vi "NEWER NEWEST Tilt Platform Controller.vi"() -> ()   [LabVIEW 2014]
uses:
  <vilib>/Utility/file.llb/Write To Spreadsheet File (DBL).vi
  <vilib>/Utility/file.llb/Read From Spreadsheet File (DBL).vi
  <vilib>/DAQmx/create/channels.llb/DAQmx Create Channel (DO-Digital Output).vi
  <vilib>/DAQmx/create/channels.llb/DAQmx Create Channel (AI-Voltage-Basic).vi
  <vilib>/DAQmx/configure/timing.llb/DAQmx Timing (Sample Clock).vi
  <vilib>/DAQmx/create/channels.llb/DAQmx Create Channel (DI-Digital Input).vi
  <vilib>/DAQmx/create/channels.llb/DAQmx Create Channel (CO-Pulse Generation-Ticks).vi
  <vilib>/DAQmx/configure/timing.llb/DAQmx Timing (Implicit).vi
  <vilib>/DAQmx/configure/trigger.llb/DAQmx Start Trigger (Digital Edge).vi
  <vilib>/DAQmx/read.llb/DAQmx Read (Analog 1D Wfm NChan NSamp).vi
  <vilib>/DAQmx/read.llb/DAQmx Read (Digital Wfm 1Chan NSamp).vi
  <vilib>/Waveform/DWDTOps.llb/DWDT Digital to Boolean Array.vi
  <vilib>/DAQmx/write.llb/DAQmx Write (Digital 1D Bool 1Chan 1Samp).vi
panel:
  out "In Position":bool
  in  "Divisor":u32=40
  in  "Signal Input":tag="/Dev3/PFI0"
  in  "Counter to Use":tag="Dev3/ctr0"
  in  "Start from Tilt":i32
  out "Ready":bool
  in  "Replay File":path=path "C:/Documents and Settings/theMaster/Desktop/Tilt Platform Control 9232015/Labview/Current_Tilts.csv"
  in  "Load Sequence":bool
  in  "Format":string="%.3f"
  in  "Delimiter":string=","
  in  "Column/Row Major":bool
  in  "Append to File?":bool=TRUE
  out "File Path":path
  out "Waveform Chart (Multiple Plots)":waveform(dbl)[](graph)
  in  "Callib Acce":bool
  in  "Callib Load Cell":bool
  in  "Transect?":bool
  in  "Week Number":dbl
  in  "Rat ID":string
  out "4":bool
  out "5":bool
  out "6":bool
  out "2":bool
  out "1":bool
  out "3":bool
  in  "Baseline Angle":dbl
  out "Angle":i32
  out "Total Force (g)":i32
  out "Completed Tilts":i32
  out "Current Tilt":i32
  out "Current ITI (s)":i32
  in  "Tirgger 6":bool=TRUE
  in  "Enable Left Slow":bool=TRUE
  in  "Enable Left Medium":bool=TRUE
  in  "Enable Left Fast":bool=TRUE
  in  "Enable Right Slow":bool=TRUE
  in  "Enable Right Medium":bool=TRUE
  in  "Enable Right Fast":bool=TRUE
  out "Left Slow":i32
  out "Left Medium":i32
  out "Left Fast":i32
  out "Right Slow":i32
  out "Right Medium":i32
  out "Right Fast":i32
  out "Practice?":bool
  in  "Stop 2":bool
  in  "Pause":bool=TRUE
  in  "Start":bool
  in  "Trial Per Tilt":dbl=3.0
  in  "ITI Base (s)":dbl=2.0 format="%#.2g"
  in  "ITI Random Multiplier":dbl=1.0 format="%#.2g"
  in  "Clock Source":i32(slide)=1 caption="Choose a setting:" scale=0.0..1.0
  # "Rat Ground Reaction Forces"
  # "Clock Source"
  # "Tilt Parameters"
  # "Animal Info"
  # "Right"
  # "Left"
  # "Current Values"
  # "Enable"
  # "Enable"
  # "Callibration"
  # "File Information"
  # "Replay Sequence"
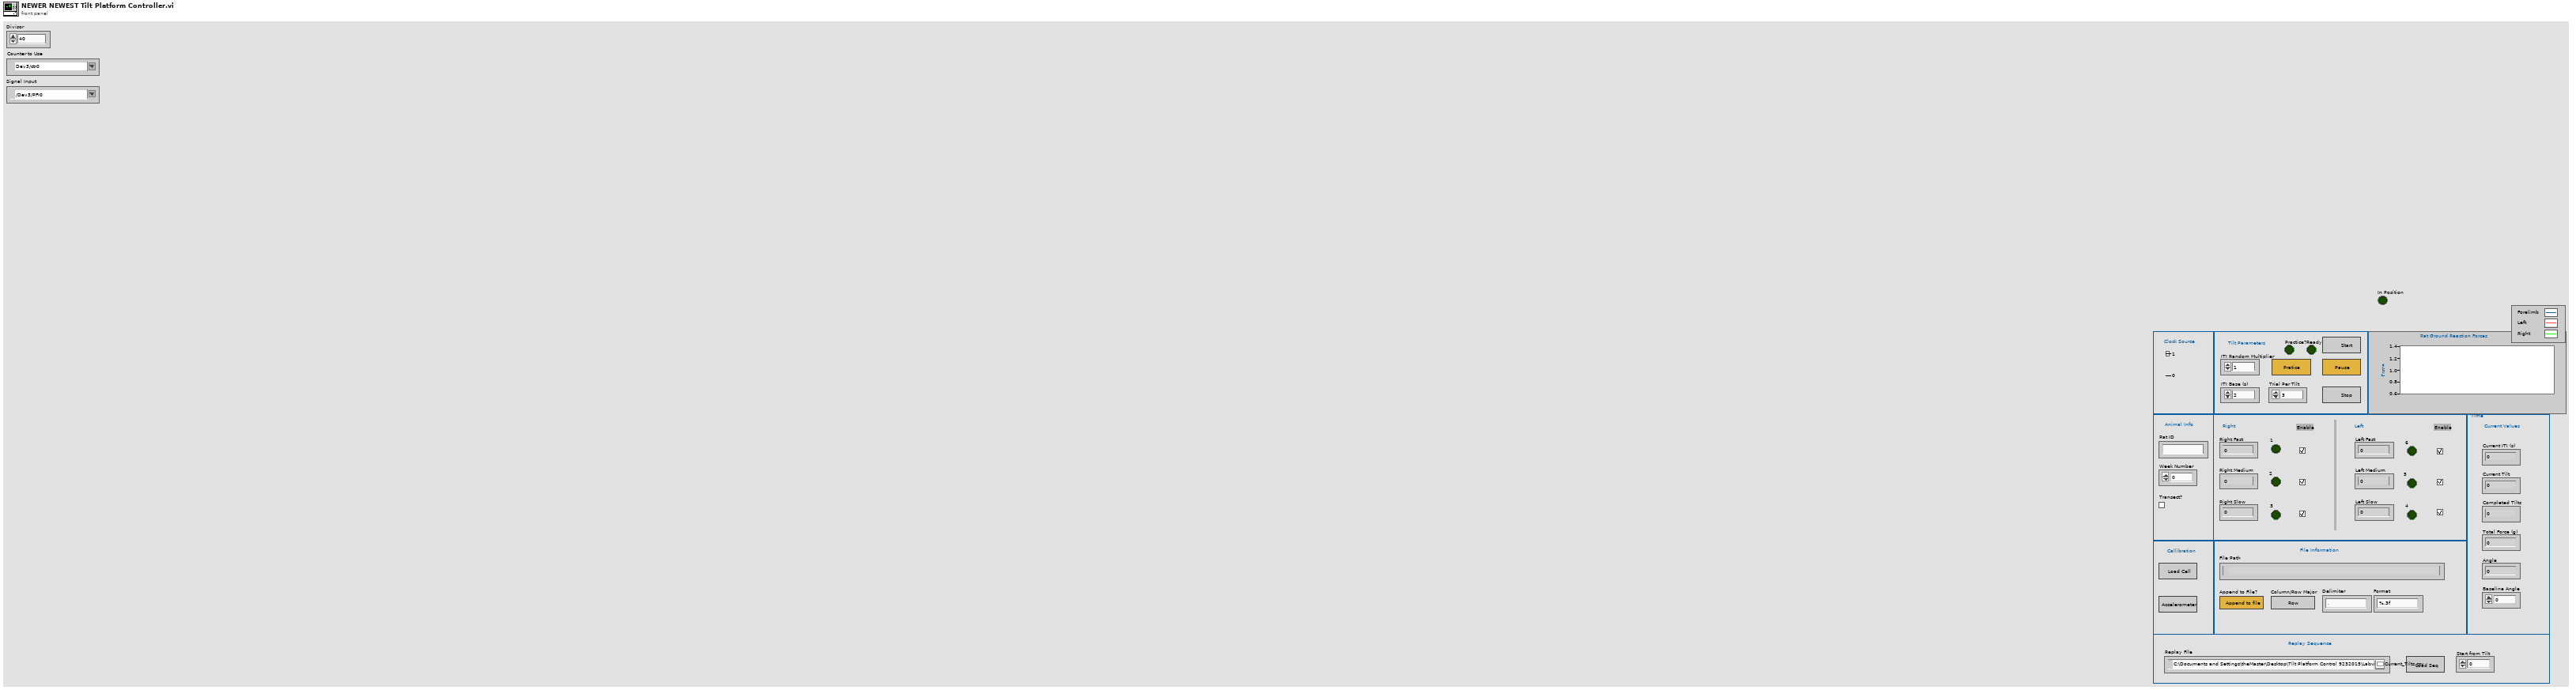
[diagram p1: front panel]
types:
  T1 = enum16{"open", "replace", "create", "open or create", "replace or create", "replace or create with confirmation"}
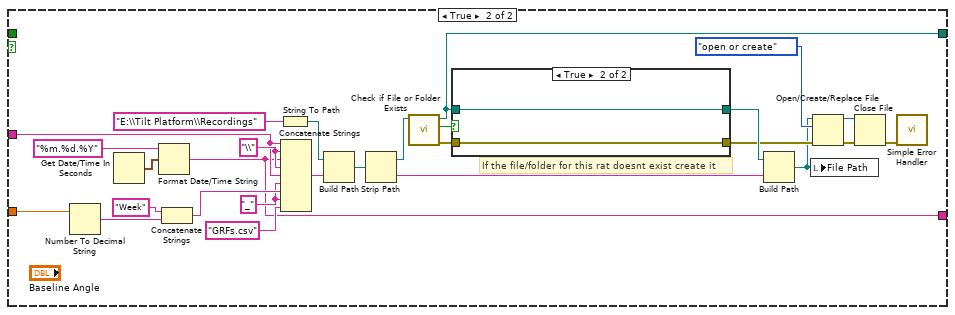
[diagram p2: hidden frame]
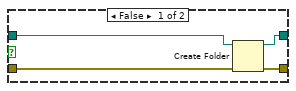
[diagram p3: hidden frame]
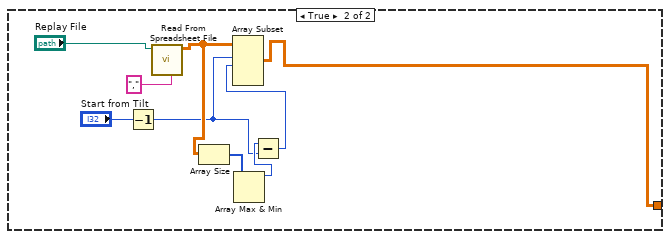
[diagram p4: hidden frame]
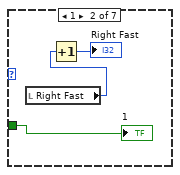
[diagram p7: hidden frame]
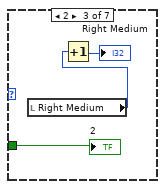
[diagram p8: hidden frame]
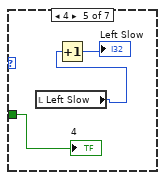
[diagram p9: hidden frame]
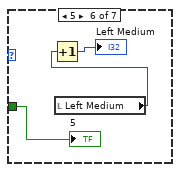
[diagram p10: hidden frame]
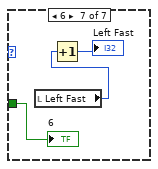
[diagram p11: hidden frame]
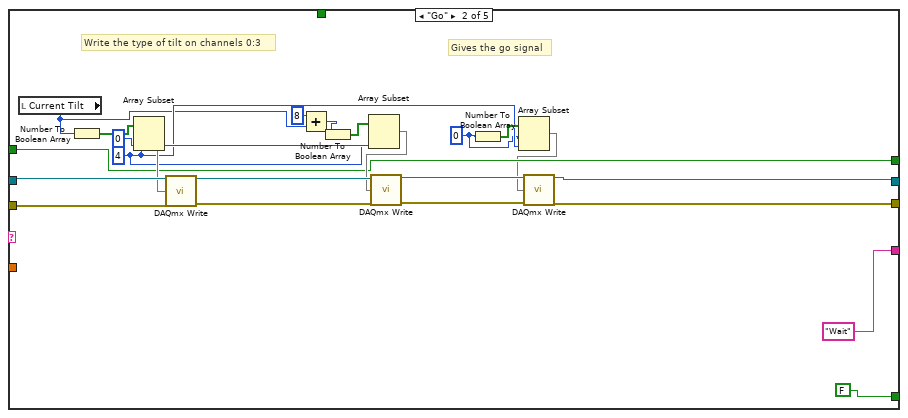
[diagram p12: hidden frame]
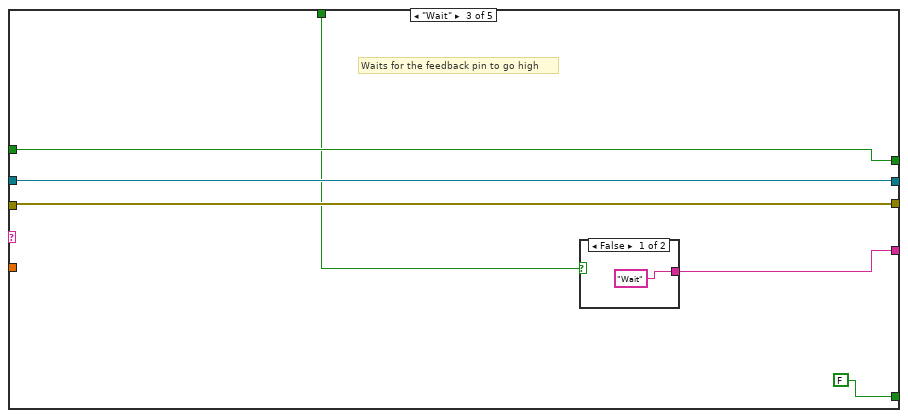
[diagram p13: hidden frame]
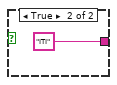
[diagram p14: hidden frame]
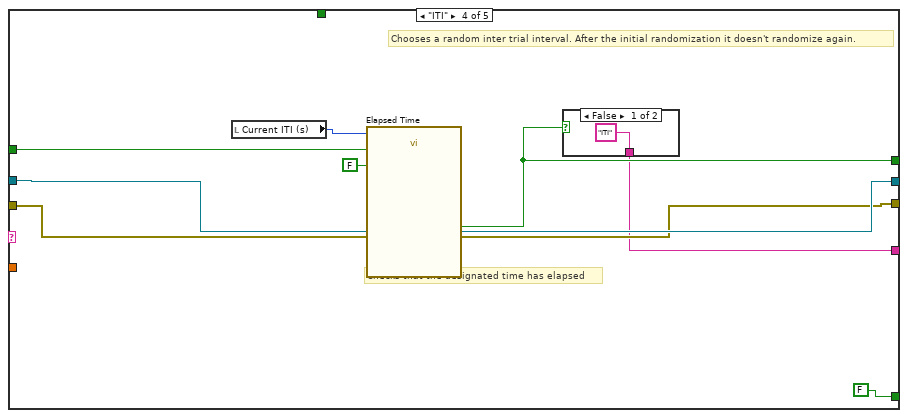
[diagram p15: hidden frame]
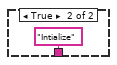
[diagram p16: hidden frame]
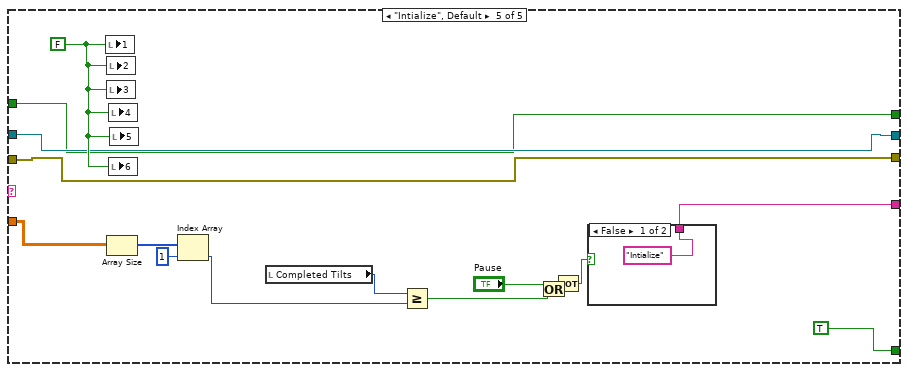
[diagram p17: hidden frame]
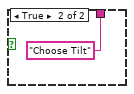
[diagram p18: hidden frame]
diagram:
  # "ai11: inclinometer output \nai16:18 are force sensor output\nai19:21 are accelerometer output\nai22: Feedback\n\nFeedback pin: P0.4"
  # "The GUI these items are not touched. Only through local variables"
  n1 = flat-sequence {
    tunnel: ["Tirgger 6"] -> w45
    tunnel: w45 -> [w50]
    tunnel: [w50] -> w44
    tunnel: [w53] -> w43
    tunnel: ["Transect?"] -> w36
    tunnel: [w47] -> w35
    tunnel: w44 -> [w90]
    tunnel: [w90] -> w42
    tunnel: w43 -> [w89]
    tunnel: [w89] -> w41
    tunnel: [w88] -> w37
    tunnel: w36 -> [w88]
    tunnel: w35 -> [w87]
    tunnel: [w87] -> w34
    tunnel: w42 -> [w94]
    tunnel: [w94] -> w22
    tunnel: [w93] -> w20
    tunnel: w41 -> [w93]
    tunnel: w37 -> [w92]
    tunnel: [w92] -> w18
    tunnel: [w91] -> w16
    tunnel: w34 -> [w91]
    tunnel: w22 -> [w98]
    tunnel: [w98] -> w21
    tunnel: w20 -> [w97]
    tunnel: [w97] -> w19
    tunnel: w18 -> [w96]
    tunnel: [w96] -> w17
    tunnel: w16 -> [w95]
    tunnel: [w95] -> w15
    tunnel: w21 -> [w105]
    tunnel: [w105] -> w33
    tunnel: w19 -> [w104]
    tunnel: [w104] -> w32
    tunnel: w17 -> [w103]
    tunnel: [w103] -> w31
    tunnel: w15 -> [w102]
    tunnel: [w102] -> w30
    tunnel: [w100] -> w14
    tunnel: [w241] -> w40
    tunnel: w33 -> [_]
    tunnel: [w234] -> w39
    tunnel: [w233] -> w38
    tunnel: w32 -> [_]
    tunnel: w31 -> [_]
    tunnel: w30 -> [_]
    tunnel: [w224] -> w29
    tunnel: [w223] -> w28
    tunnel: [w220] -> w23
    tunnel: w14 -> [w219]
    tunnel: [w219] -> w13
    tunnel: [w216] -> w12
    tunnel: [w215] -> w11
    tunnel: [w192] -> w8
    tunnel: [w191] -> w7
    tunnel: [w181] -> w4
    tunnel: [w180] -> w3
    tunnel: w40 -> [w268]
    tunnel: w39 -> [w267]
    tunnel: w38 -> [w265]
    tunnel: w29 -> [w270]
    tunnel: w28 -> [w269]
    tunnel: [w266] -> w27
    tunnel: [w264] -> w26
    tunnel: [w263] -> w25
    tunnel: [w262] -> w24
    tunnel: w23 -> [w260]
    tunnel: w13 -> [w259]
    tunnel: w12 -> [w258]
    tunnel: w11 -> [w257]
    tunnel: [w256] -> w10
    tunnel: [w255] -> w9
    tunnel: w8 -> [w253]
    tunnel: w7 -> [w254]
    tunnel: [w251] -> w6
    tunnel: [w252] -> w5
    tunnel: w4 -> [w250]
    tunnel: w3 -> [w249]
    tunnel: [w247] -> w2
    tunnel: [w246] -> w1
    tunnel: w27 -> [w433]
    tunnel: w26 -> [w432]
    tunnel: w25 -> [w431]
    tunnel: w24 -> [w430]
    tunnel: w10 -> [w428]
    tunnel: w9 -> [w429]
    tunnel: w6 -> [w423]
    tunnel: w5 -> [w424]
    tunnel: w2 -> [_]
    tunnel: w1 -> [_]
    frame #0 {
      # "Determine if this is a practice session. Causes files not to be saved"
      n2 = local write "Practice?"("Tirgger 6") -> ()
    }
    frame #1 {
      # "If the file doesnt exist create it"
      # "Save the file"
      # "If it's not a practice"
      n3 = Not(x=w50) -> (.not. x?=w49:bool)
      n4 = case shown="False" w49 {
        tunnel: "Transect?" -> [_ _]
        tunnel: "Week Number" -> [_ w58]
        tunnel: "Rat ID" -> [_ w57]
        tunnel: [_ w56] -> w53
        tunnel: [_ w54] -> w47
        frame False {
        }
        frame True {
          w59 = "_"
          w64 = "\\" ("string")
          # "If the file/folder for this rat doesnt exist create it"
          n5 = Number To Decimal String(number=w58) -> (decimal integer string=w79:string)  [unwired: 1 in]
          n6 = Get Date/Time In Seconds() -> (seconds since 1Jan1904=w76:timestamp)
          n7 = Format Date/Time String(time format string (%c)="%m.%d.%Y", seconds (now)=w76) -> (date/time string=w54:string)  [unwired: 1 in]
          n8 = Concatenate Strings("Week" ("string"), w79) -> (w63:string)
          n9 = String To Path(string="E:\\Tilt Platform\\Recordings") -> (path=w78:path)
          n10 = Concatenate Strings(w57, w64, w54, w64, w57, w59, w63, w59, "GRFs.csv" ("string")) -> (w61:string)
          n11 = Build Path(base path=w78, name or relative path=w61) -> (appended path=w74:path)
          n12 = Strip Path(path=w74) -> (stripped path=w73:path, name=w62:string)
          n13 = call <vilib>:"Check if File or Folder Exists.vi"("path"=w73) -> ("error out"=w71:errorcluster, "file or folder exists?"=w72:bool, "dup path"=w56:path)  [unwired: 8 in]
          n14 = case shown="True" w72 {
            tunnel: w56 -> [w84 w86]
            tunnel: w71 -> [w83 w85]
            tunnel: [w82 w86] -> w68
            tunnel: [w81 w85] -> w67
            frame False {
              n15 = Create Folder(path (use dialog)=w84, error in=w83) -> (created path=w82:path, error out=w81:errorcluster)  [unwired: 1 in, 1 out]
            }
            frame True {
            }
          }
          n16 = Build Path(base path=w68, name or relative path=w62) -> (appended path=w55:path)
          n17 = local write "File Path"(w55) -> ()
          n18 = Open/Create/Replace File(file path (use dialog)=w55, error in=w67, operation (0:open)=T1."open or create") -> (refnum out=w70:refnum<file>, error out=w66:errorcluster)  [unwired: 3 in, 1 out]
          n19 = Close File(refnum=w70, error in=w66) -> (error out=w65:errorcluster)  [unwired: 1 out]
          n20 = call <vilib>:"Simple Error Handler.vi"("error in (no error)"=w65) -> ()  [unwired: 4 in, 5 out]
        }
      }
    }
    frame #2 {
      # "Otherwise load the previous callibration values"
      # "Pull up sub vi"
      # "If you chose to calibrate the load cells"
    }
    frame #3 {
      # "Otherwise load the previous values"
      # "Load the sub vi"
      # "If you chose to calibrate the accelerometer"
    }
    frame #4 {
      # "This keeps the program frozen until you hit start. This way it gives you time to change anything you need to update for the tilt types"
      n21 = while {
        stop <- "Start" stop-if-true
      }
    }
    frame #5 {
      # "load cell regression params"
      # "acceleremeter regression params"
      n22 = case shown="False" "Load Sequence" {
        tunnel: [w106 w165] -> w100
        frame False {
          # "Generate an array of randomized ITI for the same size of the tilt array"
          # "Generate the array of randomized tilts"
          n23 = Boolean To (0,1)(Boolean="Enable Left Fast") -> (0, 1=w149:i16)
          n24 = Boolean To (0,1)(Boolean="Enable Left Slow") -> (0, 1=w141:i16)
          n25 = Boolean To (0,1)(Boolean="Enable Right Slow") -> (0, 1=w138:i16)
          n26 = Boolean To (0,1)(Boolean="Enable Right Medium") -> (0, 1=w133:i16)
          n27 = Boolean To (0,1)(Boolean="Enable Right Fast") -> (0, 1=w129:i16)
          n28 = Boolean To (0,1)(Boolean="Enable Left Medium") -> (0, 1=w146:i16)
          n29 = Multiply(x=w149, y=6 ("length")) -> (x*y=w143:i32)
          n30 = Multiply(x=w141, y=4 ("length")) -> (x*y=w135:i32)
          n31 = Multiply(x=w138, y=3 ("length")) -> (x*y=w134:i32)
          n32 = Multiply(x=w133, y=2 ("length")) -> (x*y=w130:i32)
          n33 = Multiply(x=w129, y=1 ("length")) -> (x*y=w126:i32)
          n34 = Multiply(x=w146, y=5 ("length")) -> (x*y=w142:i32)
          n35 = Initialize Array(w134, "Trial Per Tilt") -> (w122:i32[])
          n36 = Initialize Array(w130, "Trial Per Tilt") -> (w121:i32[])
          n37 = Initialize Array(w135, "Trial Per Tilt") -> (w123:i32[])
          n38 = Initialize Array(w142, "Trial Per Tilt") -> (w124:i32[])
          n39 = Initialize Array(w126, "Trial Per Tilt") -> (w120:i32[])
          n40 = Initialize Array(w143, "Trial Per Tilt") -> (w125:i32[])
          n41 = Build Array (concatenate)(w125, w124, w123, w122, w121, w120) -> (w118:i32[])
          n42 = for {
            tunnel: w118 -> [w162] mode=indexing
            tunnel: [w163] -> w152 mode=indexing
            n43 = Random Number (0-1)() -> (number: 0 to 1=w164:dbl)
            n44 = Bundle("number: 0 to 1"=w164, w162) -> (w163:cluster{"number: 0 to 1":dbl, i32})  [unwired: 1 in]
          }
          n45 = Sort 1D Array(array=w152) -> (sorted array=w151:cluster{"number: 0 to 1":dbl, i32}[])
          n46 = for {
            tunnel: w151 -> [w161] mode=indexing
            tunnel: [w160] -> w119 mode=indexing
            n47 = Unbundle(w161) -> (w160:i32)  [unwired: 1 out]
          }
          n48 = Current VI's Path() -> (path=w113:path)
          n49 = Strip Path(path=w113) -> (stripped path=w112:path)  [unwired: 1 out]
          n50 = for {
            tunnel: [w158] -> w107 mode=indexing if=w159
            tunnel: w119 -> [w158] mode=indexing
            n51 = Not Equal To 0?(x=w158) -> (x != 0?=w159:bool)
          }
          n52 = Array Size(array=w107) -> (size(s)=w117:i32)
          n53 = for {
            N: w117 -> [_]
            tunnel: [w153] -> w116 mode=indexing
            n54 = Random Number (0-1)() -> (number: 0 to 1=w156:dbl)
            n55 = Multiply(x="ITI Random Multiplier", y=w156) -> (x*y=w155:dbl)
            n56 = Add(x=w155, y="ITI Base (s)") -> (x+y=w153:dbl)
          }
          n57 = Build Array(w107, w116) -> (w106:dbl[][])
          n58 = Path To String(path=w112) -> (string=w111:string)
          n59 = Concatenate Strings(w111, "\\Current_Tilts.csv") -> (w109:string)
          n60 = String To Path(string=w109) -> (path=w115:path)
          n61 = call-poly <vilib>:"Write To Spreadsheet File.vi"("delimiter (\\t)"="," ("delimiter (\\t)"), "transpose? (no:F)"=TRUE, "2D data"=w106, "file path (dialog if empty)"=w115) -> ()  [unwired: 4 in, 1 out]
        }
        frame True {
          n62 = Decrement(x="Start from Tilt") -> (x-1=w166:i32)
          n63 = call-poly <vilib>:"Read From Spreadsheet File.vi"("delimiter (\\t)"="," ("delimiter (\\t)"), "file path (dialog if empty)"="Replay File") -> ("all rows"=w171:dbl[][])  [unwired: 5 in, 4 out]
          n64 = Array Size(array=w171) -> (size(s)=w170:i32[])
          n65 = Array Max & Min(array=w170) -> (max value=w168:i32)  [unwired: 3 out]
          n66 = Subtract(x=w168, y=w166) -> (x-y=w169:i32)
          n67 = Array Subset(array=w171, index (row)=w166, length (row)=w169) -> (w165:dbl[][])  [unwired: 2 in]
        }
      }
    }
    frame #6 {
      w176 = 10171 items=["Rising"=10280, "Falling"=10171] ("edge")
      w196 = 10214 items=["High"=10192, "Low"=10214] ("idle state")
      w195 = 10123 items=["Finite Samples"=10178, "Continuous Samples"=10123, "Hardware Timed Single Point"=12522] ("sample mode")
      (unwired) 10171 items=["Rising"=10280, "Falling"=10171] ("edge")
      (unwired) tag "/Dev3/PFI1" ("source")
      w221 = 10123 items=["Finite Samples"=10178, "Continuous Samples"=10123, "Hardware Timed Single Point"=12522] ("sample mode")
      w235 = 10083 items=["default"=-1, "RSE"=10083, "NRSE"=10078, "Differential"=10106, "Pseudodifferential"=12529] ("input terminal configuration")
      w227 = 1000.0 ("rate")
      # "A 2D array of tilts and ITIs from a file or generated just now"
      # "Merging the errors for  digital and analog input tasks"
      # "Using analog sample clock to get digital data"
      # "change back to 16"
      # "This is the repeated sequence array"
      n68 = Array Size(array=w219) -> (size(s)=w232:i32[])
      n69 = Greater?(x=w232, y=0) -> (0:w218:bool[])
      n70 = And Array Elements(Boolean array=w218) -> (logical AND=→"Ready":bool)
      n71 = Subtract(x="Divisor", y=u32 2 ("high ticks")) -> (x-y=w204:u32)
      n72 = case shown="0" "Clock Source" {
        tunnel: [_ tag "/Dev3/PFI2" ("source")] -> w206
        frame 1, Default {
        }
        frame 0 {
        }
      }
      n73 = call-poly <vilib>:"DAQmx Create Virtual Channel.vi"("high ticks"=u32 2, "low ticks"=w204, "counter"="Counter to Use", "source of ticks"="Signal Input", "idle state"=w196, "initial delay"=w204) -> ("task out"=w197:refnum<k21>, "error out"=w198:errorcluster)  [unwired: 8 in]
      n74 = call-poly <vilib>:"DAQmx Create Virtual Channel.vi"("lines"=tag "Dev3/port0/line4") -> ("task out"=w228:refnum<k21>, "error out"=w229:errorcluster)  [unwired: 13 in]
      n75 = call-poly <vilib>:"DAQmx Create Virtual Channel.vi"("maximum value"=10.0, "minimum value"=-10.0, "input terminal configuration"=w235, "physical channels"=tag "Dev3/ai4:6,Dev3/ai0:2,Dev3/ai3") -> ("task out"=w236:refnum<k21>, "error out"=w237:errorcluster)  [unwired: 10 in]
      n76 = call-poly <vilib>:"DAQmx Timing.vi"("task/channels in"=w197, "sample mode"=w195, "error in"=w198) -> ("task out"=w193:refnum<k21>, "error out"=w194:errorcluster)  [unwired: 11 in]
      n77 = call-poly <vilib>:"DAQmx Timing.vi"("task/channels in"=w228, "sample mode"=w221, "rate"=w227, "source"=tag "/Dev3/PFI12", "error in"=w229) -> ("task out"=w226:refnum<k21>, "error out"=w225:errorcluster)  [unwired: 9 in]
      n78 = call-poly <vilib>:"DAQmx Timing.vi"("task/channels in"=w236, "sample mode"=w221, "rate"=w227, "source"=w206, "error in"=w237) -> ("task out"=w190:refnum<k21>, "error out"=w178:errorcluster)  [unwired: 9 in]
      n79 = call <vilib>:"DAQmx Start Task.vi"("task/channels in"=w193, "error in"=w194) -> ("task out"=w192:refnum<k21>, "error out"=w191:errorcluster)  [unwired: 12 in]
      n80 = call <vilib>:"DAQmx Start Task.vi"("task/channels in"=w226, "error in"=w225) -> ("task out"=w223:refnum<k21>, "error out"=w224:errorcluster)  [unwired: 12 in]
      n81 = Current VI's Path() -> (path=w189:path)
      n82 = Strip Path(path=w189) -> (stripped path=w188:path)  [unwired: 1 out]
      n83 = call-poly <vilib>:"DAQmx Trigger.vi"("task/channels in"=w190, "source"=tag "/Dev3/PFI1", "edge"=w176, "error in"=w178) -> ("task out"=w179:refnum<k21>, "error out"=w177:errorcluster)  [unwired: 10 in]
      n84 = Path To String(path=w188) -> (string=w187:string)
      n85 = Current VI's Path() -> (path=w214:path)
      n86 = Concatenate Strings(w187, "\\Temp_Ts.csv") -> (w185:string)
      n87 = Strip Path(path=w214) -> (stripped path=w213:path)  [unwired: 1 out]
      n88 = String To Path(string=w185) -> (path=w184:path)
      n89 = Path To String(path=w213) -> (string=w212:string)
      n90 = call-poly <vilib>:"DAQmx Create Virtual Channel.vi"("lines"=tag "Dev3/port0/line0:3") -> ("task out"=w243:refnum<k21>, "error out"=w242:errorcluster)  [unwired: 13 in]
      n91 = Concatenate Strings(w212, "\\Temp_Sensor.csv") -> (w210:string)
      n92 = String To Path(string=w210) -> (path=w209:path)
      n93 = Open/Create/Replace File(file path (use dialog)=w184, operation (0:open)=T1."replace or create", access (0:read/write)=enum16{"read/write", "read-only", "write-only"}."read/write") -> (refnum out=w181:refnum<file>, error out=w180:errorcluster)  [unwired: 3 in, 1 out]
      n94 = Merge Errors(w191, w177, w224) -> (w222:errorcluster)
      n95 = call <vilib>:"DAQmx Start Task.vi"("task/channels in"=w243, "error in"=w242) -> ("task out"=w241:refnum<k21>, "error out"=w220:errorcluster)  [unwired: 12 in]
      n96 = Open/Create/Replace File(file path (use dialog)=w209, operation (0:open)=T1."replace or create", access (0:read/write)=enum16{"read/write", "read-only", "write-only"}."read/write") -> (refnum out=w216:refnum<file>, error out=w215:errorcluster)  [unwired: 3 in, 1 out]
      n97 = call <vilib>:"DAQmx Start Task.vi"("task/channels in"=w179, "error in"=w222) -> ("task out"=w234:refnum<k21>, "error out"=w233:errorcluster)  [unwired: 12 in]
    }
    frame #7 {
      # "Start the state machine with \"intialize\""
      n98 = while {
        tunnel: w270 -> [w326]
        tunnel: w269 -> [w331]
        tunnel: w268 -> [w322]
        tunnel: w260 -> [w321]
        tunnel: [w330] -> w266
        tunnel: w267 -> [w332]
        tunnel: w265 -> [w329]
        tunnel: [w328] -> w264
        tunnel: [w327] -> w263
        tunnel: [w297] -> w262
        shift-right: [w323] -> _
        shift-left: " Intialize" -> [w324]
        shift-right: [w320] -> _
        shift-left: TRUE ("Time has Elapsed") -> [w319]
        tunnel: w259 -> [w316]
        tunnel: w258 -> [w275]
        tunnel: w257 -> [w274]
        tunnel: [w292] -> w256
        tunnel: [w291] -> w255
        tunnel: w254 -> [w290]
        tunnel: w253 -> [w289]
        tunnel: [w288] -> w251
        tunnel: [w287] -> w252
        tunnel: w250 -> [_]
        tunnel: w249 -> [_]
        tunnel: [w272] -> w247
        tunnel: [w271] -> w246
        stop <- w318 stop-if-true
        (unwired) "0"
        (unwired) "1"
        (unwired) FALSE ("prepend array or string size? (T)")
        # "Plot only load cells"
        # "convert all the waveforms read into a data array then convert into string to write to file"
        # "Use an OR statement to concatinate the 10 digital signals read"
        # "Read in 10 samples per iteration for both analog and digital data"
        # "The program can only end if its we're in the intialize stage"
        # "Currrent state"
        # "Reset for ITI timer"
        # "Feedback from motor signalling tilt complete"
        # "Current Tilt"
        # "Update the count for a given tilt type"
        # "Right Fast = 1\nRight Mid = 2\nRight Slow = 3\nLeft Fast = 4\nLeft Mid = 5\nLeft Slow = 6"
        # "Stops the loop"
        # "Digital input"
        # "Analog input"
        # "Digital output"
        n99 = call-poly <vilib>:"DAQmx Read.vi"("task/channels in"=w332, "number of samples per channel"=100, "error in"=w329) -> ("task out"=w330:refnum<k21>, "data"=w296:waveform(dbl)[], "error out"=w328:errorcluster)  [unwired: 10 in]
        n100 = Array Subset(array=w296, index=0, length=3) -> (→"Waveform Chart (Multiple Plots)":waveform(dbl)[])
        n101 = call-poly <vilib>:"DAQmx Read.vi"("task/channels in"=w331, "number of samples per channel"=-1, "error in"=w326) -> ("task out"=w327:refnum<k21>, "data"=w278:digitalwaveform, "error out"=w297:errorcluster)  [unwired: 10 in]
        n102 = call <vilib>:"DAQmx Is Task Done.vi"("task/channels in"=w289, "error in"=w290) -> ("task out"=w288:refnum<k21>, "error out"=w287:errorcluster)  [unwired: 11 in, 1 out]
        n103 = call-poly <vilib>:"Digital to Boolean Array.vi"("digital waveform"=w278) -> ("boolean array"=w277:bool[][])  [unwired: 9 in, 1 out]
        n104 = And Array Elements(Boolean array=w277) -> (logical AND=w276:bool)
        "In Position" <- w276
        n105 = case shown="\"Choose Tilt\"" w324 {
          tunnel: ["Go" "Wait" w391 w399 w419] -> w323
          tunnel: w322 -> [w345 w386 w393 w402 w418]
          tunnel: w321 -> [w344 w385 w392 w401 w417]
          tunnel: [w345 w374 w393 w402 w418] -> w292
          tunnel: [w344 w373 w392 w401 w417] -> w291
          tunnel: [w343 w377 w390 w400 w416] -> w320
          tunnel: w319 -> [w343 w377 w390 w398 w416]
          tunnel: [FALSE FALSE FALSE FALSE TRUE] -> w317
          tunnel: w316 -> [w340 _ _ _ w414]
          tunnel: w276 -> [_ _ w388 _ _]
          frame "Choose Tilt" {
            # "Turn on the LED for the chosen tilt"
            # "Update the current ITI and tilt values"
            # "This has just one Tilt and ITI"
            # "We select the top most index from the array"
            # "This array has the tilt & ITI"
            # "Build an array where the disabled tilt types are set to zero"
            n106 = local read "Completed Tilts"() -> (w333:i32)
            n107 = Index Array(array=w340, index (col)=w333) -> (element=w339:dbl[])  [unwired: 1 in]
            n108 = Index Array(array=w339, index #1=0 ("index"), index #2=1 ("index")) -> (element #1=w336:dbl, element #2=→"Current ITI (s)":dbl)
            "Current Tilt" <- w336
            n109 = Increment(x=w333) -> (x+1=→"Completed Tilts":i32)
            n110 = case shown="3" w336 {
              tunnel: TRUE -> [_ w347 w350 w353 w356 w359 w362]
              frame Default {
              }
              frame 1 {
                n111 = local read "Right Fast"() -> (w348:i32)
                n112 = Increment(x=w348) -> (x+1=→"Right Fast":i32)
                "1" <- w347
              }
              frame 2 {
                n113 = local read "Right Medium"() -> (w351:i32)
                n114 = Increment(x=w351) -> (x+1=→"Right Medium":i32)
                "2" <- w350
              }
              frame 3 {
                n115 = local read "Right Slow"() -> (w354:i32)
                n116 = Increment(x=w354) -> (x+1=→"Right Slow":i32)
                "3" <- w353
              }
              frame 4 {
                n117 = local read "Left Slow"() -> (w357:i32)
                n118 = Increment(x=w357) -> (x+1=→"Left Slow":i32)
                "4" <- w356
              }
              frame 5 {
                n119 = local read "Left Medium"() -> (w360:i32)
                n120 = Increment(x=w360) -> (x+1=→"Left Medium":i32)
                "5" <- w359
              }
              frame 6 {
                n121 = local read "Left Fast"() -> (w363:i32)
                n122 = Increment(x=w363) -> (x+1=→"Left Fast":i32)
                "6" <- w362
              }
            }
          }
          frame "Go" {
            w365 = u8 0
            w370 = 4 ("length")
            w379 = 0 ("index")
            # "Gives the go signal"
            # "Write the type of tilt on channels 0:3"
            n123 = local read "Current Tilt"() -> (w366:i32)
            n124 = Number To Boolean Array(number=w366) -> (Boolean array=w382:bool[])
            n125 = Array Subset(array=w382, index=w379, length=w370) -> (w381:bool[])
            n126 = call-poly <vilib>:"DAQmx Write.vi"("task/channels in"=w386, "data"=w381, "error in"=w385) -> ("task out"=w384:refnum<k21>, "error out"=w383:errorcluster)  [unwired: 10 in, 1 out]
            n127 = Add(x=u8 8, y=w366) -> (x+y=w368:i32)
            n128 = Number To Boolean Array(number=w368) -> (Boolean array=w380:bool[])
            n129 = Array Subset(array=w380, index=w379, length=w370) -> (w378:bool[])
            n130 = call-poly <vilib>:"DAQmx Write.vi"("task/channels in"=w384, "data"=w378, "error in"=w383) -> ("task out"=w376:refnum<k21>, "error out"=w375:errorcluster)  [unwired: 10 in, 1 out]
            n131 = Number To Boolean Array(number=w365) -> (Boolean array=w372:bool[])
            n132 = Array Subset(array=w372, index=w365, length=w370) -> (w371:bool[])
            n133 = call-poly <vilib>:"DAQmx Write.vi"("task/channels in"=w376, "data"=w371, "error in"=w375) -> ("task out"=w374:refnum<k21>, "error out"=w373:errorcluster)  [unwired: 10 in, 1 out]
          }
          frame "Wait" {
            # "Waits for the feedback pin to go high"
            n134 = case shown="False" w388 {
              tunnel: ["Wait" "ITI"] -> w391
              frame False {
              }
              frame True {
              }
            }
          }
          frame "ITI" {
            # "Checks that the designated time has elapsed"
            # "Chooses a random inter trial interval. After the initial randomization it doesn't randomize again."
            n135 = local read "Current ITI (s)"() -> (w396:i32)
            n136 = call "Elapsed Time"("Time Target (s)"=w396, "Reset"=w398, "Auto Reset"=FALSE) -> ("Time has Elapsed"=w400:bool)  [unwired: 9 in, 7 out]
            n137 = case shown="False" w400 {
              tunnel: ["ITI" "Intialize"] -> w399
              frame False {
              }
              frame True {
              }
            }
          }
          frame "Intialize", Default {
            w420 = FALSE
            n138 = local write "1"(w420) -> ()
            n139 = local write "2"(w420) -> ()
            n140 = local write "3"(w420) -> ()
            n141 = Array Size(array=w414) -> (size(s)=w413:i32[])
            n142 = local write "4"(w420) -> ()
            n143 = local write "6"(w420) -> ()
            n144 = local write "5"(w420) -> ()
            n145 = Index Array(array=w413, index=1) -> (element=w411:i32)
            n146 = local read "Completed Tilts"() -> (w410:i32)
            n147 = Greater Or Equal?(x=w410, y=w411) -> (x >= y?=w408:bool)
            n148 = Or(x="Pause", y=w408) -> (x .or. y?=w409:bool)
            n149 = Not(x=w409) -> (.not. x?=w407:bool)
            n150 = case shown="False" w407 {
              tunnel: ["Intialize" "Choose Tilt"] -> w419
              frame False {
              }
              frame True {
              }
            }
          }
        }
        n151 = Index Array(array=w296, index #1=0 ("number of samples per channel"), index #2=1 ("number of samples per channel"), index #3=2 ("number of samples per channel"), index #4=3 ("number of samples per channel"), index #5=4 ("number of samples per channel"), index #6=5 ("number of samples per channel"), index #7=6 ("number of samples per channel")) -> (element #1=w308:waveform(dbl), element #2=w307:waveform(dbl), element #3=w306:waveform(dbl), element #4=w305:waveform(dbl), element #5=w304:waveform(dbl), element #6=w303:waveform(dbl), element #7=w302:waveform(dbl))
        n152 = Unbundle By Name(w308) -> ("Y"=w286:dbl[])
        n153 = Unbundle By Name(w307) -> ("Y"=w285:dbl[])
        n154 = Unbundle By Name(w306) -> ("Y"=w284:dbl[])
        n155 = Unbundle By Name(w305) -> ("Y"=w283:dbl[])
        n156 = Unbundle By Name(w304) -> ("Y"=w282:dbl[])
        n157 = Unbundle By Name(w303) -> ("Y"=w281:dbl[])
        n158 = Unbundle By Name(w302) -> ("Y"=w280:dbl[])
        n159 = Build Array(w286, w285, w284, w283, w282, w281, w280) -> (w299:dbl[][])
        n160 = Transpose 2D Array(2D array=w299) -> (transposed array=w298:dbl[][])
        n161 = Array To Spreadsheet String(delimiter (Tab)=",", array=w298, 3:"%3f" ("format string")) -> (spreadsheet string=w273:string)
        n162 = Write to Text File(file (use dialog)=w275, text=w273, error in=w274) -> (refnum out=w272:refnum<file>, error out=w271:errorcluster)  [unwired: 1 in, 1 out]
        n163 = local read "Stop 2"() -> (w318:bool)
        n164 = And(x=w317, y=w318) -> ()  [unwired: 1 out]
      }
    }
    frame #8 {
      # "Clear digital ouput tasks"
      # "accelerometer regression params"
      # "load cell regression params"
      # "Perform post processing here:"
      # "Clear digital input task"
      # "Clear analog input task"
      # "Clear digital output task"
      # "Resets all values once program ends"
      n165 = call <vilib>:"DAQmx Clear Task.vi"("task in"=w431, "error in"=w430) -> ()  [unwired: 13 in, 1 out]
      n166 = call <vilib>:"DAQmx Clear Task.vi"("task in"=w428, "error in"=w429) -> ()  [unwired: 13 in, 1 out]
      n167 = call <vilib>:"DAQmx Clear Task.vi"("task in"=w433, "error in"=w432) -> ()  [unwired: 13 in, 1 out]
      n168 = call <vilib>:"DAQmx Stop Task.vi"("task/channels in"=w423, "error in"=w424) -> ("task out"=w427:refnum<k21>, "error out"=w426:errorcluster)  [unwired: 12 in]
      n169 = call <vilib>:"DAQmx Clear Task.vi"("task in"=w427, "error in"=w426) -> ("error out"=w425:errorcluster)  [unwired: 13 in]
      n170 = call <vilib>:"Simple Error Handler.vi"("error in (no error)"=w425) -> ()  [unwired: 4 in, 5 out]
      n171 = control-ref of="This VI"() -> (w436:refnum<vi>)
      n172 = invoke class="VI" method="Default Vals.Reinit All"(reference=w436) -> (reference out=w434:refnum<vi>, error out=w435:errorcluster)  [unwired: 2 in, 1 out]
      n173 = Close Reference(reference=w434, error in (no error)=w435) -> ()  [unwired: 1 out]
    }
  }
